vi "Shooter.vi"(1 "Shooter Power":dbl, 2 "Enable Shooter":bool) -> ()   [LabVIEW 2016]
uses:
  Robot Global Data.vi
  <vilib>/Rock Robotics/Network Tables/NT Write Number.vi
panel:
  out "RPM 3":dbl
  out "RPM 2":dbl
  out "RPM":dbl
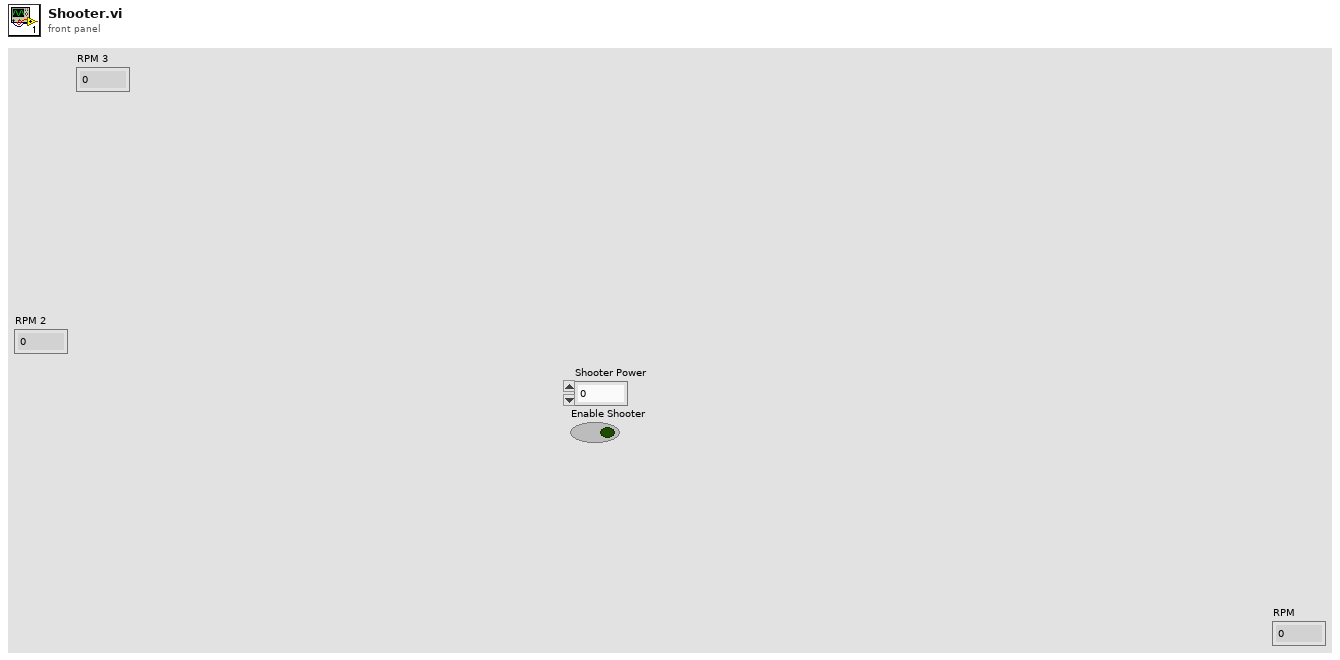
[diagram p1: front panel]
types:
  T1 = typedef "WPI_MotorControlDeviceRef.ctl" = cluster{"DeviceStatus":errorcluster, "Type":T2, "PWM":cluster{"PWM Channel":T3, "DeadBand":T4}, "CAN":cluster{"Device Number":u8, "SetOutput VI Ref":variant, "GetOutput VI Ref":variant, "Enable VI Ref":variant, "Disable VI Ref":variant, "Data":variant}, "Invert":bool}
  T2 = typedef "WPI_MotorControlType.ctl" = enum16{"PWM", "CAN"}
  T3 = typedef "FPGA_DIOPWMChannel.ctl" = enum8{"PWM 0", "PWM 1", "PWM 2", "PWM 3", "PWM 4", "PWM 5", "PWM 6", "PWM 7", "PWM 8", "PWM 9", "PWM MXP 0", "PWM MXP 1", "PWM MXP 2", "PWM MXP 3", "PWM MXP 4", "PWM MXP 5", "PWM MXP 6", "PWM MXP 7", "PWM MXP 8", "PWM MXP 9", "Invalid"}
  T4 = typedef "WPI_PWMDeadband.ctl" = cluster{"Name":string, "maxPositivePwm":i32, "minPositivePwm":i32, "centerPwm":i32, "maxNegativePwm":i32, "minNegativePwm":i32, "angularRange":u16}
  T5 = typedef "WPI_AnalogChannelDevRef.ctl" = cluster{"DevStatus":errorcluster, "Analog Channel":T6}
  T6 = typedef "FPGA_AIChannel.ctl" = enum8{"AI 0", "AI 1", "AI 2", "AI 3", "AI MXP 0", "AI MXP 1", "AI MXP 2", "AI MXP 3", "Invalid"}
  T7 = typedef "WPI_DigitalInputDevRef.ctl" = cluster{"DevStatus":errorcluster, "DIO Channel":T8}
  T8 = typedef "FPGA_DIOChannel.ctl" = enum8{"DIO 0", "DIO 1", "DIO 2", "DIO 3", "DIO 4", "DIO 5", "DIO 6", "DIO 7", "DIO 8", "DIO 9", "DIO MXP 0", "DIO MXP 1", "DIO MXP 2", "DIO MXP 3", "DIO MXP 4", "DIO MXP 5", "DIO MXP 6", "DIO MXP 7", "DIO MXP 8", "DIO MXP 9", "DIO MXP 10", "DIO MXP 11", "DIO MXP 12", "DIO MXP 13", "DIO MXP 14", "DIO MXP 15", "SPI Port CS1", "SPI Port CS2", "SPI Port CS3", "SPI Port MISO", "SPI Port MOSI", "Invalid"}
  T9 = typedef "WPI_CANTalonSRX_GlobalStatus.ctl" = cluster{"Applied Throttle":dbl, "Module Enabled":bool, "CAN Error":errorcluster, "Closed Loop Error":dbl, "Forward Limit Switch Closed":bool, "Reverse Limit Switch Closed":bool, "Sensor Position":dbl, "Sensor Velocity":dbl, "Current":dbl, "Sticky Fault - Over Temp":bool, "Sticky Fault - Under Voltage":bool, "Sticky Fault - Forward Limit":bool, "Sticky Fault - Reverse Limit":bool, "Sticky Fault - Forward Soft Limit":bool, "Sticky Fault - Reverse Soft Limit":bool, "Brake is Enabled":bool, "Encoder Position":dbl, "Encoder Velocity":dbl, "Encoder Index Count":dbl, "Encoder A Pin State":bool, "Encoder B Pin State":bool, "Encoder Index Pin State":bool, "Analog In":dbl, "Analog In Velocity":dbl, "Temperature (C)":dbl, "Battery Voltage":dbl, "Control 5 Is Supported":bool, "Current Profile Slot Select":dbl, "Pos Div 8":bool, "Vel Div 4":bool, "Pulse Width Position":i32, "Pulse Width Velocity":i32, "Pulse Width Rise To Rise (us)":i32, "Pulse Width Rise To Fall (us)":i32, "Mot Prof Active Is Under Run":bool, "Mot Prof Active Has Under Run":bool, "Mot Prof Active Is Last":bool, "Mot Prof Active Velocity Only":bool, "Mot Prof Active Is Valid":bool, "Mot Prof Buffer Is Full":bool, "Mot Prof Active Profile Slot Select":i32, "Mot Prof NextID":i32, "Mot Prof Count":i32, "Mot Prof Active Velocity":dbl, "Mot Prof Active Position":dbl, "Mot Prof Output Enable":i32}
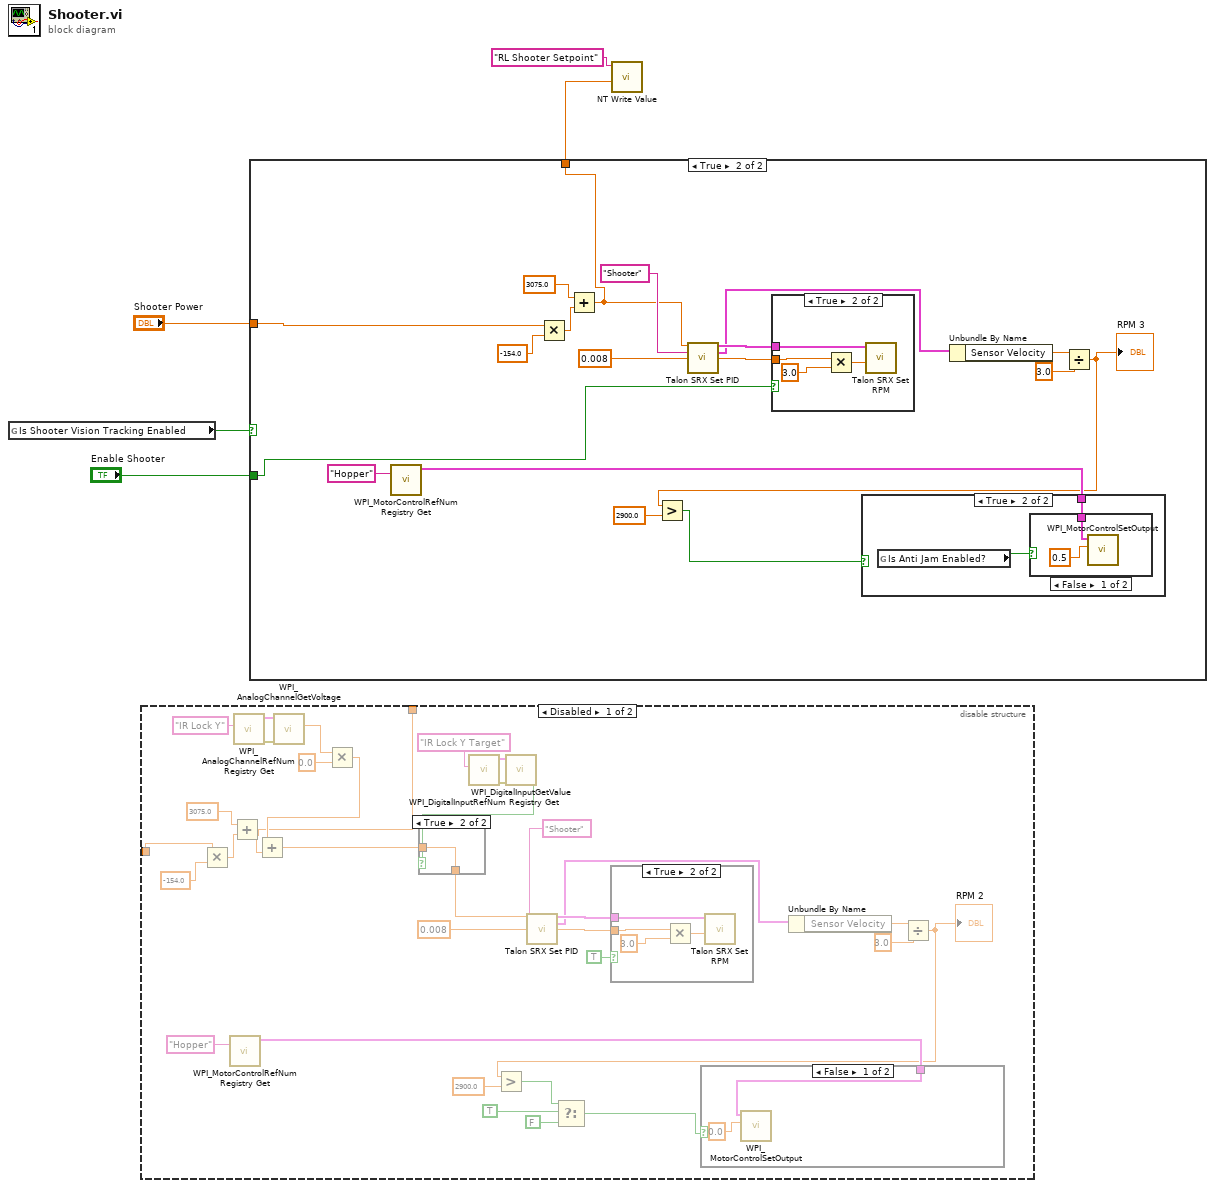
[diagram p0: block diagram]
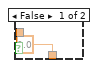
[diagram p2: hidden frame]
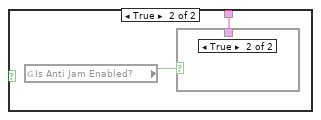
[diagram p3: hidden frame]
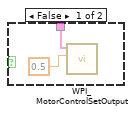
[diagram p4: hidden frame]
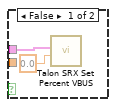
[diagram p5: hidden frame]
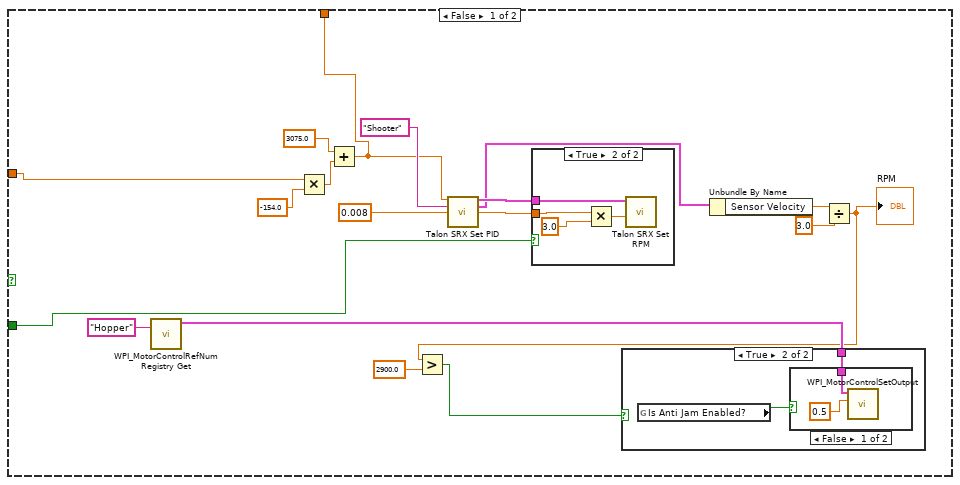
[diagram p7: hidden frame]
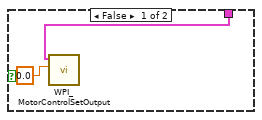
[diagram p8: hidden frame]
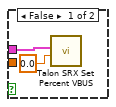
[diagram p10: hidden frame]
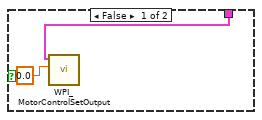
[diagram p11: hidden frame]
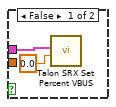
[diagram p13: hidden frame]
diagram:
  n1 = global read "Robot Global Data.vi" "Is Shooter Vision Tracking Enabled"() -> (w5:bool)
  n2 = disable-structure shown="Disabled" {
    disable-tunnel: _ -> [w9 _]
    disable-tunnel: [w6 _] -> _
    frame Disabled {
      n3 = Multiply(x=w9, y=-154.0) -> (x*y=w22:dbl)
      n4 = call <vilib>:"WPI_MotorControlRefNum Registry Get.vi"("refnum name"="Hopper") -> ("MotorControlDevRef"=w33:T1)  [unwired: 9 in, 1 out]
      n5 = Add(x=3075.0 ("Target RPM"), y=w22) -> (x+y=w6:dbl)
      n6 = call <vilib>:"WPI_AnalogChannelRefNum Registry Get.vi"("refnum name"="IR Lock Y") -> ("error out"=w14:errorcluster, "AIDeviceRef"=w15:T5)  [unwired: 9 in]
      n7 = call <vilib>:"WPI_AnalogChannelGetVoltage.vi"("error in (no error)"=w14, "AIDeviceRef"=w15) -> ("Voltage"=w11:dbl)  [unwired: 7 in, 2 out]
      n8 = Multiply(x=w11, y=0.0) -> (x*y=w10:dbl)
      n9 = Add(x=w10, y=w6) -> (x+y=w20:dbl)
      n10 = call <vilib>:"WPI_DigitalInputRefNum Registry Get.vi"("refnum name"="IR Lock Y Target") -> ("error out"=w18:errorcluster, "DigitalInputDevRef"=w19:T7)  [unwired: 9 in]
      n11 = call <vilib>:"WPI_DigitalInputGetValue.vi"("error in (no error)"=w18, "DigitalInputDevRef"=w19) -> ("Value"=w16:bool)  [unwired: 7 in, 2 out]
      n12 = case shown="True" w16 {
        tunnel: [0.0 w40] -> w21
        tunnel: w20 -> [_ w40]
        frame False {
        }
        frame True {
        }
      }
      n13 = call "Talon SRX Set PID.vi"("Target RPM"=w21, "Talon SRX Refnum Name"="Shooter", "P"=0.008) -> ("CAN Talon SRX Ref"=w37:T1, "Talon SRX Status"=w32:T9, "Target RPM Output"=w36:dbl)  [unwired: 9 in, 1 out]
      n14 = case shown="True" TRUE {
        tunnel: w37 -> [w48 w51]
        tunnel: w36 -> [_ w49]
        frame False {
          n15 = call "Talon SRX Set Percent VBUS.vi"("Desired VBus"=0.0, "CAN Talon SRX Ref"=w48) -> ()  [unwired: 10 in]
        }
        frame True {
          n16 = Multiply(x=w49, y=3.0) -> (x*y=w50:dbl)
          n17 = call "Talon SRX Set RPM.vi"("Desired RPM"=w50, "CAN Talon SRX Ref"=w51) -> ()  [unwired: 10 in]
        }
      }
      n18 = Unbundle By Name(w32) -> ("Sensor Velocity"=w31:dbl)
      n19 = Divide(x=w31, y=3.0) -> (x/y=w27:dbl)
      "RPM 2" <- w27
      n20 = Greater?(x=w27, y=2900.0) -> (0:w28:bool)
      n21 = Select(t=w28, s=TRUE, f=FALSE) -> (s? t:f=w29:bool)
      n22 = case shown="False" w29 {
        tunnel: w33 -> [w41 w43]
        frame False {
          n23 = call <vilib>:"WPI_MotorControlSetOutput.vi"("Output"=0.0, "MotorControlDevRef"=w41) -> ()  [unwired: 7 in, 3 out]
        }
        frame True {
          n24 = global read "Robot Global Data.vi" "Is Anti Jam Enabled?"() -> (w44:bool)
          n25 = case shown="True" w44 {
            tunnel: w43 -> [w45 _]
            frame False {
              n26 = call <vilib>:"WPI_MotorControlSetOutput.vi"("Output"=0.5, "MotorControlDevRef"=w45) -> ()  [unwired: 7 in, 3 out]
            }
            frame True {
            }
          }
        }
      }
    }
    frame Enabled {
    }
  }
  n27 = case shown="True" w5 {
    tunnel: "Enable Shooter" -> [w56 w85]
    tunnel: "Shooter Power" -> [w55 w84]
    tunnel: [w54 w83] -> w1
    frame False {
      n28 = call <vilib>:"WPI_MotorControlRefNum Registry Get.vi"("refnum name"="Hopper") -> ("MotorControlDevRef"=w65:T1)  [unwired: 9 in, 1 out]
      n29 = Multiply(x=w55, y=-154.0) -> (x*y=w57:dbl)
      n30 = Add(x=3075.0 ("Target RPM"), y=w57) -> (x+y=w54:dbl)
      n31 = call "Talon SRX Set PID.vi"("Target RPM"=w54, "Talon SRX Refnum Name"="Shooter", "P"=0.008) -> ("CAN Talon SRX Ref"=w69:T1, "Talon SRX Status"=w64:T9, "Target RPM Output"=w68:dbl)  [unwired: 9 in, 1 out]
      n32 = case shown="True" w56 {
        tunnel: w69 -> [w78 w81]
        tunnel: w68 -> [_ w79]
        frame False {
          n33 = call "Talon SRX Set Percent VBUS.vi"("Desired VBus"=0.0, "CAN Talon SRX Ref"=w78) -> ()  [unwired: 10 in]
        }
        frame True {
          n34 = Multiply(x=w79, y=3.0) -> (x*y=w80:dbl)
          n35 = call "Talon SRX Set RPM.vi"("Desired RPM"=w80, "CAN Talon SRX Ref"=w81) -> ()  [unwired: 10 in]
        }
      }
      n36 = Unbundle By Name(w64) -> ("Sensor Velocity"=w63:dbl)
      n37 = Divide(x=w63, y=3.0) -> (x/y=w61:dbl)
      "RPM" <- w61
      n38 = Greater?(x=w61, y=2900.0) -> (0:w53:bool)
      n39 = case shown="True" w53 {
        tunnel: w65 -> [w71 w73]
        frame False {
          n40 = call <vilib>:"WPI_MotorControlSetOutput.vi"("Output"=0.0, "MotorControlDevRef"=w71) -> ()  [unwired: 7 in, 3 out]
        }
        frame True {
          n41 = global read "Robot Global Data.vi" "Is Anti Jam Enabled?"() -> (w74:bool)
          n42 = case shown="False" w74 {
            tunnel: w73 -> [w75 _]
            frame False {
              n43 = call <vilib>:"WPI_MotorControlSetOutput.vi"("Output"=0.5, "MotorControlDevRef"=w75) -> ()  [unwired: 7 in, 3 out]
            }
            frame True {
            }
          }
        }
      }
    }
    frame True {
      n44 = call <vilib>:"WPI_MotorControlRefNum Registry Get.vi"("refnum name"="Hopper") -> ("MotorControlDevRef"=w95:T1)  [unwired: 9 in, 1 out]
      n45 = Multiply(x=w84, y=-154.0) -> (x*y=w87:dbl)
      n46 = Add(x=3075.0 ("Target RPM"), y=w87) -> (x+y=w83:dbl)
      n47 = call "Talon SRX Set PID.vi"("Target RPM"=w83, "Talon SRX Refnum Name"="Shooter", "P"=0.008) -> ("CAN Talon SRX Ref"=w99:T1, "Talon SRX Status"=w94:T9, "Target RPM Output"=w98:dbl)  [unwired: 9 in, 1 out]
      n48 = case shown="True" w85 {
        tunnel: w99 -> [w108 w111]
        tunnel: w98 -> [_ w109]
        frame False {
          n49 = call "Talon SRX Set Percent VBUS.vi"("Desired VBus"=0.0, "CAN Talon SRX Ref"=w108) -> ()  [unwired: 10 in]
        }
        frame True {
          n50 = Multiply(x=w109, y=3.0) -> (x*y=w110:dbl)
          n51 = call "Talon SRX Set RPM.vi"("Desired RPM"=w110, "CAN Talon SRX Ref"=w111) -> ()  [unwired: 10 in]
        }
      }
      n52 = Unbundle By Name(w94) -> ("Sensor Velocity"=w93:dbl)
      n53 = Divide(x=w93, y=3.0) -> (x/y=w91:dbl)
      "RPM 3" <- w91
      n54 = Greater?(x=w91, y=2900.0) -> (0:w86:bool)
      n55 = case shown="True" w86 {
        tunnel: w95 -> [w101 w103]
        frame False {
          n56 = call <vilib>:"WPI_MotorControlSetOutput.vi"("Output"=0.0, "MotorControlDevRef"=w101) -> ()  [unwired: 7 in, 3 out]
        }
        frame True {
          n57 = global read "Robot Global Data.vi" "Is Anti Jam Enabled?"() -> (w104:bool)
          n58 = case shown="False" w104 {
            tunnel: w103 -> [w105 _]
            frame False {
              n59 = call <vilib>:"WPI_MotorControlSetOutput.vi"("Output"=0.5, "MotorControlDevRef"=w105) -> ()  [unwired: 7 in, 3 out]
            }
            frame True {
            }
          }
        }
      }
    }
  }
  n60 = call-poly <vilib>:"NT Write Value.vi"("Numeric"=w1, "Name"="RL Shooter Setpoint") -> ()  [unwired: 9 in, 1 out]
